vi "LIMIT_LINE Save.vi"(11 "data":variant) -> ()   [LabVIEW 2020]
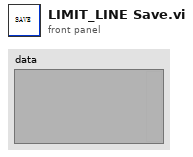
[diagram p1: front panel]
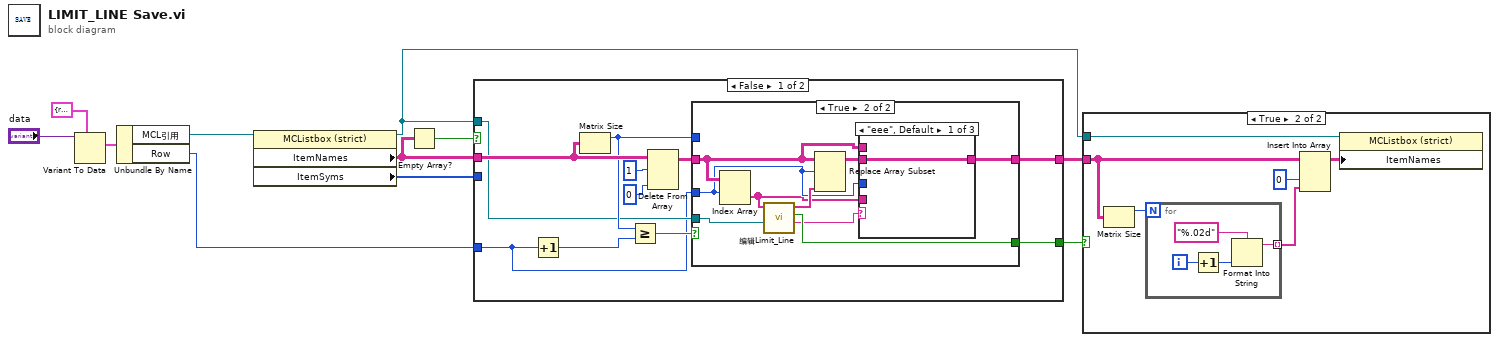
[diagram p0: block diagram]
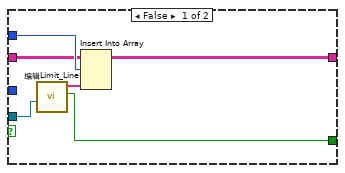
[diagram p3: hidden frame]
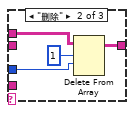
[diagram p4: hidden frame]
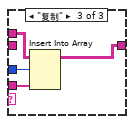
[diagram p5: hidden frame]
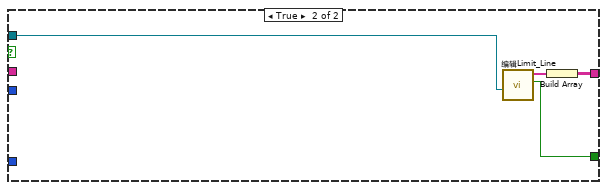
[diagram p6: hidden frame]
diagram:
  n1 = Variant To Data(type=cluster{"MCL引用":refnum<vi>, "Row":i32} {"MCL引用"=refnum, "Row"=0}, Variant="data") -> (data=w3:cluster{"MCL引用":refnum<vi>, "Row":i32})  [unwired: 1 in, 1 out]
  n2 = Unbundle By Name(w3) -> ("MCL引用"=w1:refnum<vi>, "Row"=w2:i32)
  n3 = property class="MCListbox (strict)"(reference=w1) -> (reference out=w5:refnum<vi>, "ItemNames"=w9:string[][], "ItemSyms"=w6:i32[])  [unwired: 1 in, 1 out]
  n4 = Empty Array?(array=w9) -> (empty?=w10:bool)
  n5 = case shown="False" w10 {
    tunnel: [w17 w49] -> w8
    tunnel: w9 -> [w22 _]
    tunnel: w2 -> [w12 _]
    tunnel: [w18 w48] -> w7
    tunnel: w6 -> [_ _]
    tunnel: w5 -> [w14 w47]
    frame False {
      n6 = Increment(x=w12) -> (x+1=w13:i32)
      n7 = Matrix Size(0:w22) -> (1:w16:i32)  [unwired: 1 out]
      n8 = Greater Or Equal?(x=w16, y=w13) -> (x >= y?=w19:bool)
      n9 = Delete From Array(array=w22, length=1 ("长度"), index (col)=0 ("禁用的索引 (列)")) -> (array with subset deleted=w15:string[][])  [unwired: 1 in, 1 out]
      n10 = case shown="True" w19 {
        tunnel: [w28 w37] -> w18
        tunnel: w15 -> [w26 w33]
        tunnel: w16 -> [w27 _]
        tunnel: [w24 w32] -> w17
        tunnel: w12 -> [_ w31]
        tunnel: w14 -> [w23 w29]
        frame False {
          n11 = call "编辑Limit_Line.vi"("引用"=w23) -> ("OK？"=w28:bool, "Data Out"=w25:string[])  [unwired: 8 in, 1 out]
          n12 = Insert Into Array(array=w26, index (row)=w27, new element=w25) -> (w24:string[][])  [unwired: 1 in]
        }
        frame True {
          n13 = Index Array(array=w33, index (row)=w31) -> (element=w30:string[])  [unwired: 1 in]
          n14 = call "编辑Limit_Line.vi"("引用"=w29, "Data In"=w30) -> ("Operate"=w35:string, "OK？"=w37:bool, "Data Out"=w36:string[])  [unwired: 7 in]
          n15 = Replace Array Subset(array=w33, new element=w36, index (row)=w31) -> (w34:string[][])  [unwired: 1 in]
          n16 = case shown="\"eee\", Default" w35 {
            tunnel: w34 -> [w38 _ _]
            tunnel: w33 -> [_ w42 w46]
            tunnel: [w38 w39 w45] -> w32
            tunnel: w31 -> [_ w40 w44]
            tunnel: w30 -> [_ _ w43]
            frame "eee", Default {
            }
            frame "删除" {
              n17 = Delete From Array(array=w42, length=1 ("长度"), index (row)=w40) -> (array with subset deleted=w39:string[][])  [unwired: 1 in, 1 out]
            }
            frame "复制" {
              n18 = Insert Into Array(array=w46, index (row)=w44, new element=w43) -> (w45:string[][])  [unwired: 1 in]
            }
          }
        }
      }
    }
    frame True {
      n19 = call "编辑Limit_Line.vi"("引用"=w47) -> ("OK？"=w48:bool, "Data Out"=w50:string[])  [unwired: 8 in, 1 out]
      n20 = Build Array(w50) -> (w49:string[][])
    }
  }
  n21 = case shown="True" w7 {
    tunnel: w5 -> [_ w56]
    tunnel: w8 -> [_ w54]
    frame False {
    }
    frame True {
      n22 = Matrix Size(0:w54) -> (1:w55:i32)  [unwired: 1 out]
      n23 = for {
        N: w55 -> [_]
        tunnel: [w57] -> w52 mode=indexing
        i -> [w59]
        n24 = Increment(x=w59) -> (x+1=w58:i32)
        n25 = Format Into String(format string="%.02d" ("格式字符串"), w58) -> (resulting string=w57:string)  [unwired: 2 in, 1 out]
      }
      n26 = Insert Into Array(array=w54, index (col)=0 ("禁用的索引 (列)"), new element=w52) -> (w51:string[][])  [unwired: 1 in]
      n27 = property class="MCListbox (strict)"(reference=w56, "ItemNames"=w51) -> ()  [unwired: 1 in, 2 out]
    }
  }
